vi "DiffDriveTrainSim_GetLeftCurrentDrawAmps.vi"(11 "DiffDriveTrainSim":T1 {"m_Motor"."Jr_KgM2" format="%13.5p"; "m_Motor"."L_H" format="%13.5p"; "m_Motor"."Kt_NMPerAmp" format="%13.5p"; "m_Motor"."KvINV_RadPerSecPerVolt" format="%13.5p"; "m_Motor"."R_Ohms" format="%13.5p"; "m_Motor"."FreeSpeed_RadPerSec" format="%13.5p"; "m_Motor"."FreeCurrent_Amps" format="%13.5p"; "m_Motor"."StallCurrent_Amps" format="%13.5p"; "m_Motor"."StallTorque_NM" format="%13.5p"; "m_Motor"."nominalVoltage_Volts" format="%13.5p"}) -> (3 "LeftCurrentDraw_Amps":dbl)   [LabVIEW 2019, in "Trajectory_Library.lvlib"]
doc: "Get the current draw of the left side of the drivetrain.\n \nInputs:\n - DiffDriveTraimSim -- Data cluster\n\nOutputs:\n - LeftCurrentDraw_Amp -- the drivetrain's left side current draw, in amps"
uses:
  Trajectory_Library.lvlib
  DIFF_DRIVE_TRAIN_SIM.ctl
  LINEAR_SYSTEM.ctl
  <vilib>/Analysis/Matrix/Datatypes/RealMatrix.ctl
  DCMOTOR.CTL
  DIFF_DRIVE_TRAIN_SIM_STATE_ENUM.ctl
  <vilib>/Analysis/Matrix/NI_Matrix.lvlib
panel:
  # "<States, 1>"
  # "<Outputs, 1>"
  # "<Inputs, 1>"
  # "<Outputs, 1>"
  # "<States,States>"
  # "<States,Inputs>"
  # "<Outputs,States>"
  # "<Outputs,Inputs>"
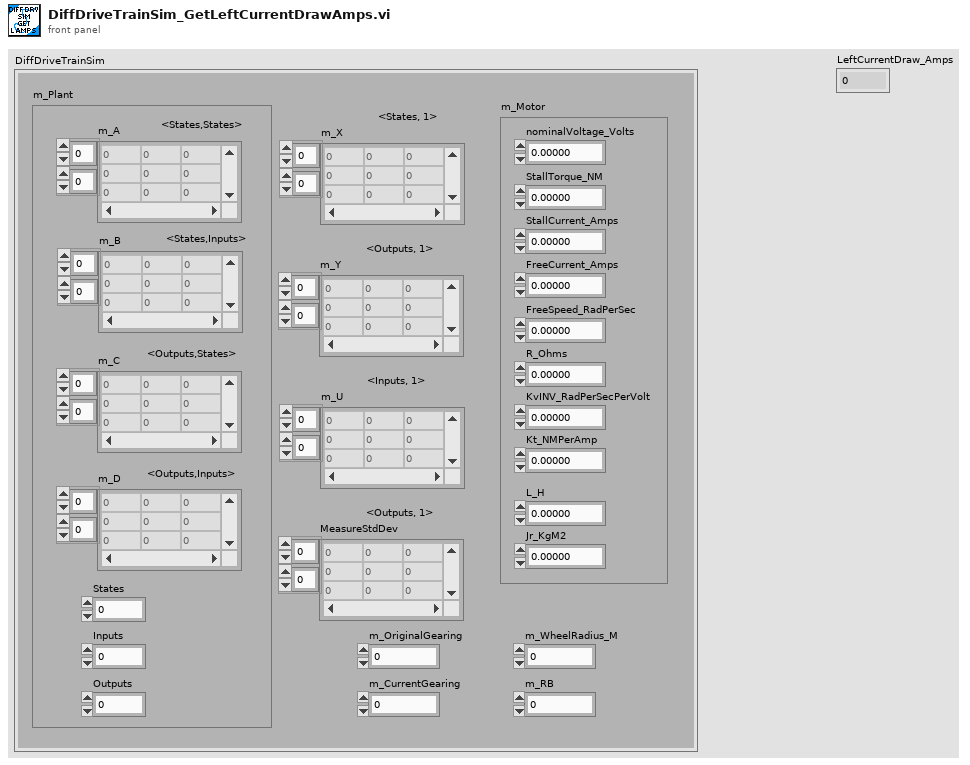
[diagram p1: front panel]
types:
  T1 = typedef "Trajectory_Library.lvlib/DIFF_DRIVE_TRAIN_SIM.ctl" = cluster{"m_Plant":T2, "m_X":T3, "m_Y":T3, "m_U":T3, "MeasureStdDev":T3, "m_Motor":T4, "m_OriginalGearing":dbl, "m_CurrentGearing":dbl, "m_WheelRadius_M":dbl, "m_RB":dbl}
  T2 = typedef "Trajectory_Library.lvlib/LINEAR_SYSTEM.ctl" = cluster{"m_A":T3, "m_B":T3, "m_C":T3, "m_D":T3, "States":i32, "Inputs":i32, "Outputs":i32}
  T3 = typedef "NI_Matrix.lvlib/RealMatrix.ctl" = dbl[][]
  T4 = typedef "Trajectory_Library.lvlib/DCMOTOR.CTL" = cluster{"nominalVoltage_Volts":dbl, "StallTorque_NM":dbl, "StallCurrent_Amps":dbl, "FreeCurrent_Amps":dbl, "FreeSpeed_RadPerSec":dbl, "R_Ohms":dbl, "KvINV_RadPerSecPerVolt":dbl, "Kt_NMPerAmp":dbl, "L_H":dbl, "Jr_KgM2":dbl}
  T5 = typedef "Trajectory_Library.lvlib/DIFF_DRIVE_TRAIN_SIM_STATE_ENUM.ctl" = enum16{"X_POS", "Y_POS", "HEADING", "LEFT_VEL", "RIGHT_VEL", "LEFT_DIST", "RIGHT_DIST"}
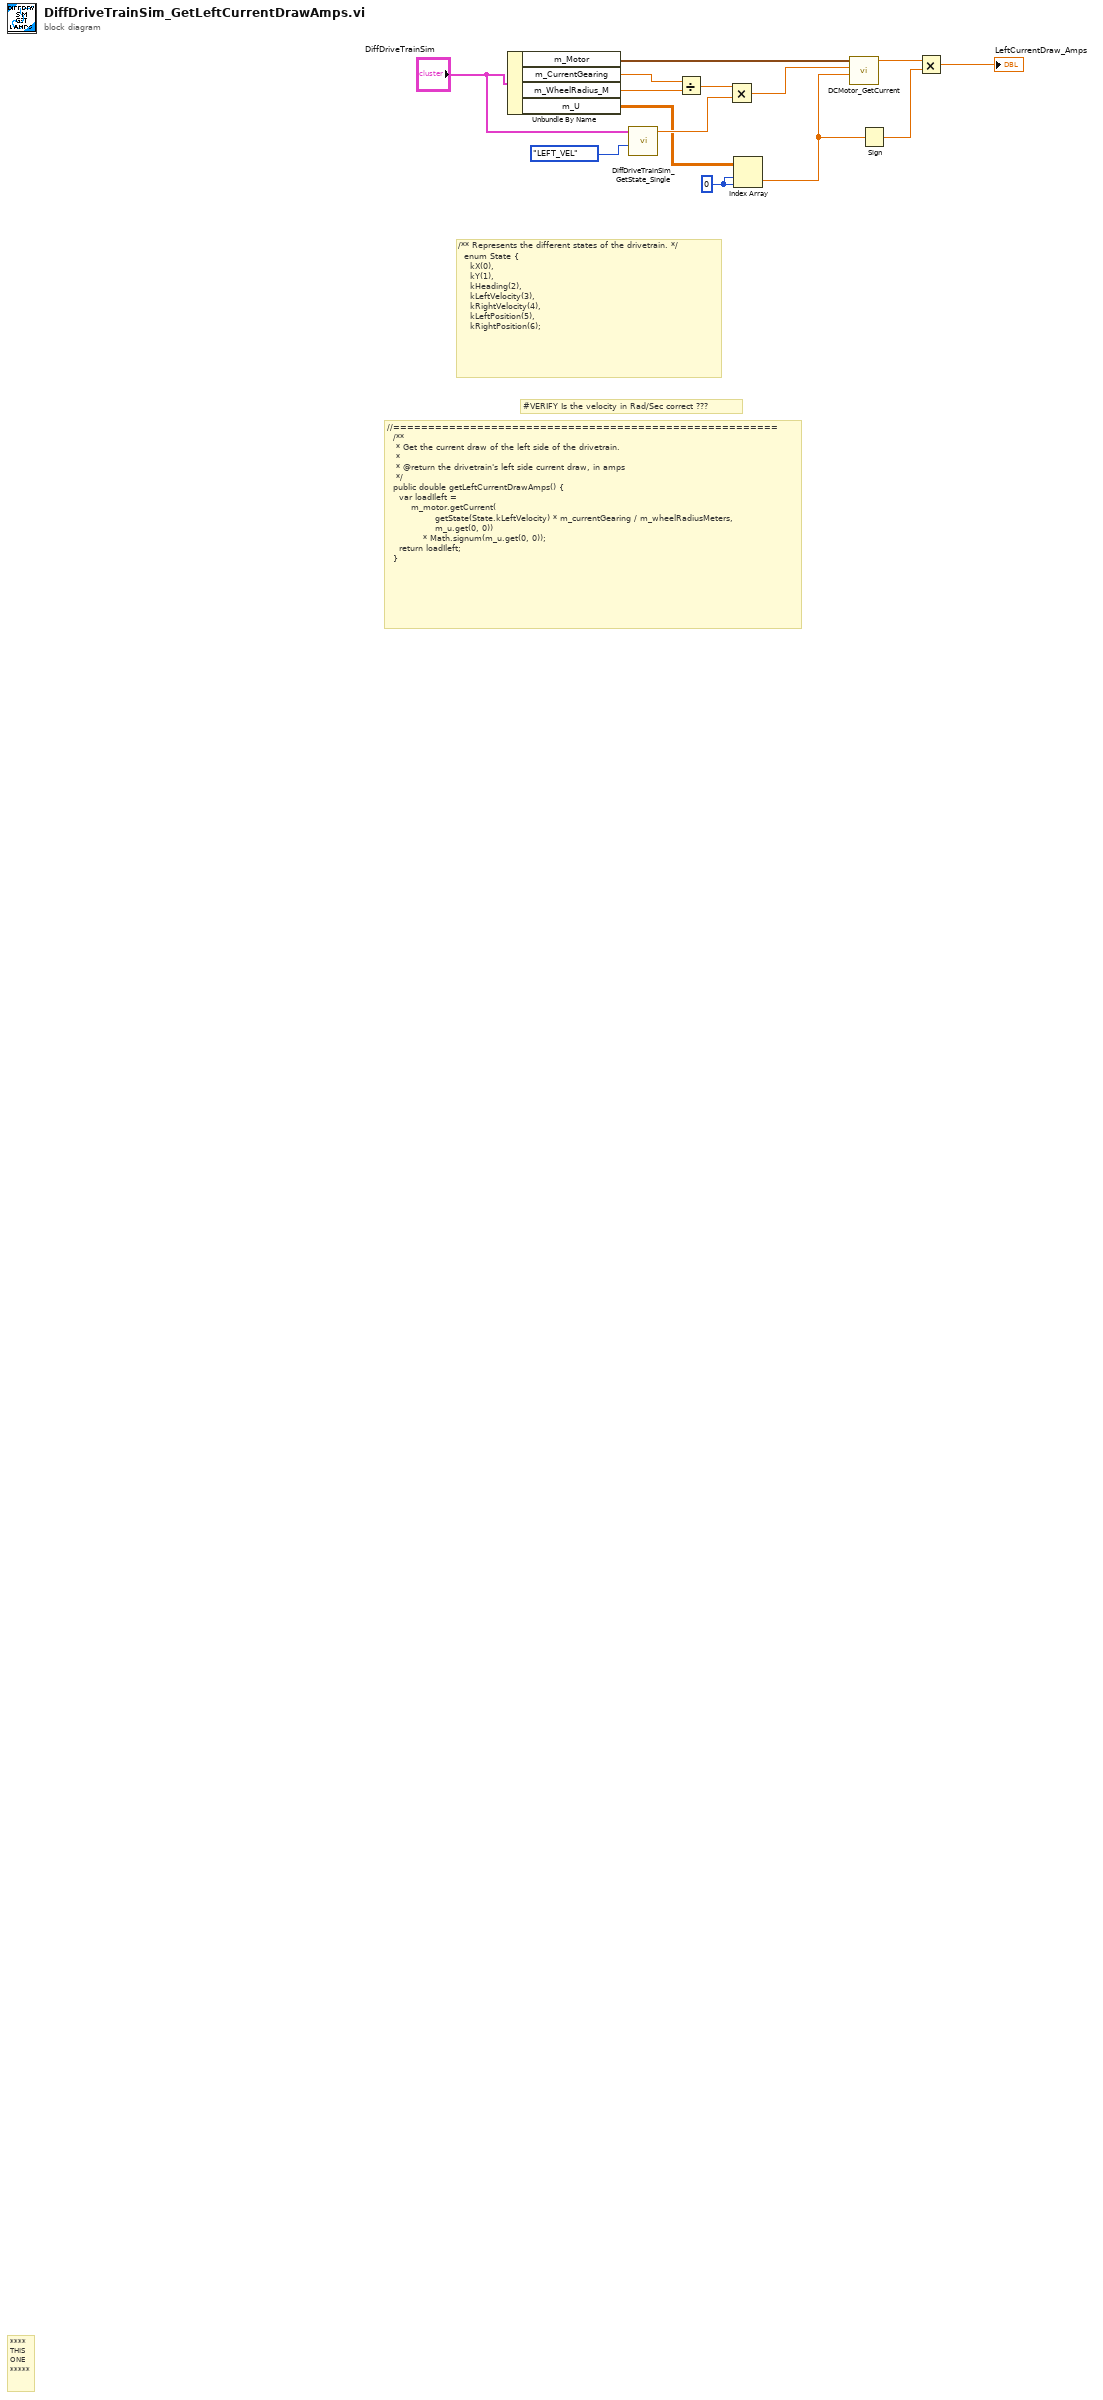
[diagram p0: block diagram]
diagram:
  w6 = 0 ("index (row)")
  # "#VERIFY Is the velocity in Rad/Sec correct ???"
  # "/** Represents the different states of the drivetrain. */\n  enum State {\n    kX(0),\n    kY(1),\n    kHeading(2),\n    kLeftVelocity(3),\n    kRightVelocity(4),\n    kLeftPosition(5),\n    kRightPosition(6);"
  # "//=======================================================\n  /**\n   * Get the current draw of the left side of the drivetrain.\n   *\n   * @return the drivetrain's left side current draw, in amps\n   */\n  public double getLeftCurrentDrawAmps() {\n    var loadIleft =\n        m_motor.getCurrent(\n                getState(State.kLeftVelocity) * m_currentGearing / m_wheelRadiusMeters,\n                m_u.get(0, 0))\n            * Math.signum(m_u.get(0, 0));\n    return loadIleft;\n  }"
  # "****\nTHIS\nONE\n*****"
  n1 = Unbundle By Name("DiffDriveTrainSim") -> ("m_Motor"=w14:T4, "m_CurrentGearing"=w13:dbl, "m_WheelRadius_M"=w12:dbl, "m_U"=w7:T3)
  n2 = call "DiffDriveTrainSim_GetState_Single.vi"("Row"=DIFF_DRIVE_TRAIN_SIM_STATE_ENUM."LEFT_VEL" ("DIFF_DRIVE_TRAIN_SIM_STATE"), "DiffDriveTrainSim"="DiffDriveTrainSim") -> ("State"=w9:dbl)  [unwired: 9 in]
  n3 = Divide(x=w13, y=w12) -> (x/y=w10:dbl)
  n4 = Multiply(x=w10, y=w9) -> (x*y=w8:dbl)
  n5 = Index Array(array=w7, index (row)=w6, index (col)=w6) -> (element=w5:dbl)
  n6 = call "DCMotor_GetCurrent.vi"("VoltageInput_Volts"=w5, "Speed_RadPerSec"=w8, "DCMOTOR"=w14) -> ("Current_Amps"=w4:dbl)  [unwired: 8 in]
  n7 = Sign(1:w5) -> (0:w3:dbl)
  n8 = Multiply(x=w4, y=w3) -> (x*y=→"LeftCurrentDraw_Amps":dbl)
